vi "Memory.Pointer.Create.vi"(8 "error in (no error)":errorcluster) -> (0 "error out":errorcluster, 3 "Pointer out":refnum<class "Memory.Pointer.lvclass">)   [LabVIEW 2016, in "LabVIEW Memory Manager.lvlib" / "Memory.Pointer.lvclass"]
uses:
  Memory.Pointer.lvclass
  Memory.Pointer.lvclass/Memory.Pointer.ctl
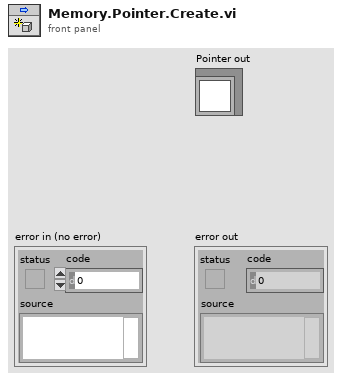
[diagram p1: front panel]
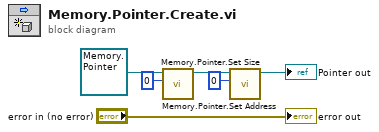
[diagram p0: block diagram]
diagram:
  n1 = call "Memory.Pointer.Set Address.vi"("address"=u64 0, "Pointer in"=refnum<class "Memory.Pointer.lvclass"> refnum ("LabVIEW Memory Manager.lvlib:Pointer")) -> ("Pointer out"=w6:refnum<class "Memory.Pointer.lvclass">)  [unwired: 8 in, 1 out]
  n2 = call "Memory.Pointer.Set Size.vi"("size"=i64 0, "Pointer in"=w6) -> ("Pointer out"=→"Pointer out":refnum<class "Memory.Pointer.lvclass">)  [unwired: 8 in, 1 out]
  "error out" <- "error in (no error)"
